vi "Narrowband Filtering - DFD.vi"() -> ()   [LabVIEW 2023]
doc: "Demonstrates how to design a narrowband FIR filter using VIs in the LabVIEW Digital Filter Design Toolkit."
uses:
  <vilib>/addons/Digital Filter Design/_Objects.llb/DFD Phase Setting.ctl
  <vilib>/addons/Digital Filter Design/NI_DigFilterLicensed.lvlib
panel:
  out "Error Message":string
  out "magnitude response":cluster{dbl, dbl, dbl[]}(graph)={0.0, 19.53125, []}
  out "phase response":cluster{dbl, dbl, "Unwrapped Phase":dbl[]}(graph)={0.0, 19.53125, "Unwrapped Phase"=[]}
  in  "filter type":T1(ring)
  in  "center freq":dbl min=0.0 format="%0.2f"
  in  "attenuation (db)":dbl=60.0 min=0.0 format="%0.1f"
  in  "ripple":dbl=0.01 min=0.0 format="%0.4f"
  in  "passband":dbl=100.0 min=0.0 format="%0.4f"
  in  "sampling freq":dbl=10000.0 min=0.0 format="%0.2f"
  in  "stopband":dbl=200.0 min=0.0 format="%0.4f"
  # "Select Help»Show Context Help and move the cursor over the VI icon for more information."
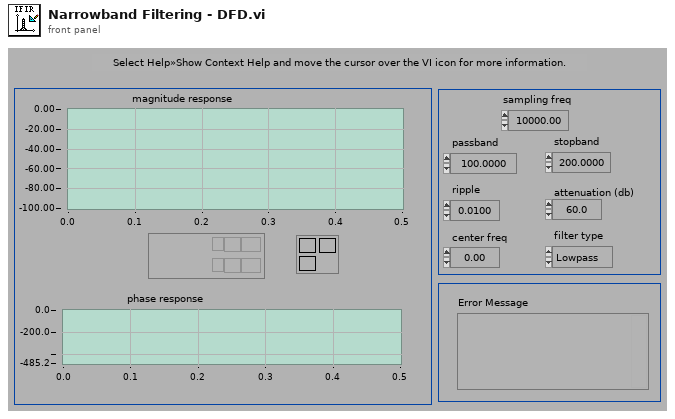
[diagram p1: front panel]
types:
  T1 = enum32{"Lowpass", "Highpass", "Bandpass", "Bandstop"}
  T2 = typedef "NI_DigFilterLicensed.lvlib/DFD Phase Setting.ctl" = cluster{"unwrap? (F)":bool, "degree? (F)":bool}
  T3 = typedef "NI_DigFilterLicensed.lvlib/DFD Filter Frequence Specification (Design).ctl" = cluster{"fpass 1":dbl, "fstop 1":dbl, "fpass 2 ":dbl, "fstop 2":dbl}
  T4 = typedef "NI_DigFilterLicensed.lvlib/DFD Narrowband Filter Obj.ctl" = cluster{"multirate filters":T5[], "filter type":enum32{"Lowpass", "Highpass", "Bandpass", "Bandstop", "Wideband-Lowpass", "Wideband-Highpass"}}
  T5 = typedef "NI_DigFilterLicensed.lvlib/DFD Multirate Filter Obj.ctl" = cluster{"mMRate_Structure":enum16{"CIC", "FIR", "IIR", "Lattice"}, "mMRate_Mode":T6, "mMRate_Factor":i32, "mMRate_FIRParams":cluster{"mMRate_FIR_H":dbl[], "mMRate_FIR_IsNyquist?":bool, "mMRate_FIR_IsSymmetric?":bool}, "mMRate_CICParams":cluster{"mMRate_CIC_#Stage":i32, "mMRate_CIC_Lag":i32, "mMRate_CIC_Type":enum16{"Lowpass", "Highpass"}}, "mMRate_Order":i32, "mMRate_Version":string, "mMRate_Comments":string, "mMRate_RationalFactor":cluster{"mMRate_L":i32, "mMRate_M":i32}, "mMRate_Fs":dbl, "mMRate_Quantized?":bool, "mMRate_QFilterGain":dbl, "mMRate_CoefWl":i16, "mMRate_Scaling":cluster{"mMRate_ScaleByPowerOf2?":bool, "mMRate_ScaleType":T7}, "mMRate_InputWl":i16, "mMRate_OutputWl":i16, "mMRate_OutputMode":T8, "mMRate_MultMode":T9, "mMRate_BitPruning":bool, "mMRate_GainWl":i16, "mMRate_OutputFwl":i16, "mMRate_SumIwl":i16, "mMRate_InputIwl ":i16, "mMRate_SumWl":i16, "mMRate_CoefIwl":i16}
  T6 = typedef "NI_DigFilterLicensed.lvlib/DFD Multirate Mode.ctl" = i16
  T7 = typedef "NI_DigFilterLicensed.lvlib/DFD Coef Norm Type.ctl" = enum16{"No Norm", "Time Domain 1-Norm", "Time Domain 2-Norm", "Time Domain Inf-Norm"}
  T8 = typedef "NI_DigFilterLicensed.lvlib/DFD Round-off Mode.ctl" = enum16{"Nearest", "Truncation"}
  T9 = typedef "NI_DigFilterLicensed.lvlib/DFD FXP MRate Multiply Mode.ctl" = enum16{"Truncated", "Full"}
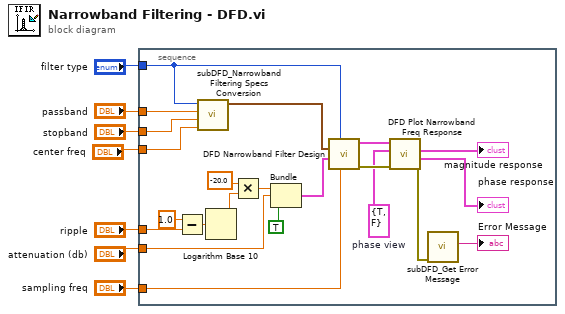
[diagram p0: block diagram]
diagram:
  n1 = stacked-sequence {
    tunnel: "sampling freq" -> [w29]
    tunnel: "passband" -> [w14]
    tunnel: "attenuation (db)" -> [w28]
    tunnel: "ripple" -> [w24]
    tunnel: "stopband" -> [w13]
    tunnel: "center freq" -> [w12]
    tunnel: "filter type" -> [w15]
    frame #0 {
      w16 = T2 {"unwrap? (F)"=TRUE, "degree? (F)"=FALSE}  # phase view
      n2 = Subtract(x=1.0, y=w24) -> (x-y=w25:dbl)
      n3 = call "subDFD_Narrowband Filtering Specs Conversion.vi"("center freq"=w12, "stopband"=w13, "passband"=w14, "filter type"=w15) -> ("freq specs [Hz]"=w11:T3)  [unwired: 7 out]
      n4 = Logarithm Base 10(1:w25) -> (0:w22:dbl)
      n5 = Multiply(x=-20.0, y=w22) -> (x*y=w20:dbl)
      n6 = Bundle(w20, "attenuation (db)"=w28, TRUE) -> (w27:cluster{dbl, "attenuation (db)":dbl, bool})  [unwired: 1 out]
      n7 = call <vilib>:"DFD Narrowband Filter Design.vi"("fs [Hz]"=w29, "filter type"=w15, "ripple specs"=w27, "freq specs [Hz]"=w11) -> ("error out"=w19:errorcluster, "narrowband filter out"=w10:T4)  [unwired: 1 in, 5 out]
      n8 = call <vilib>:"DFD Plot Narrowband Freq Response.vi"("error in (no error)"=w19, "phase view"=w16, "narrowband filter in"=w10) -> ("error out"=w8:errorcluster, "phase response"=→"phase response":cluster{"f0":dbl, "df":dbl, "phase":dbl[]}, "magnitude response"=→"magnitude response":cluster{"f0":dbl, "df":dbl, "magnitude":dbl[]})  [unwired: 3 in, 3 out]
      n9 = call <vilib>:"subDFD_Get Error Message.vi"("error in (no error)"=w8) -> ("Error Message"=→"Error Message":string)  [unwired: 10 out]
    }
  }
